vi "File.Search for Files or Folders, List Move or Copy.vi"(4 "Filter List":string, 6 "Destination Path":path, 7 "Files(F)/Folders(T)":bool, 8 "error in":errorcluster, 9 "Filters(Contain)":string[](array[string]), 10 "Action":enum16{"List", "Move", "Copy"}(ring), 11 "Source Paths":path[](array[path])) -> (0 "error out":errorcluster, 3 "Found Items":path[](array[path]))   [LabVIEW 2018]
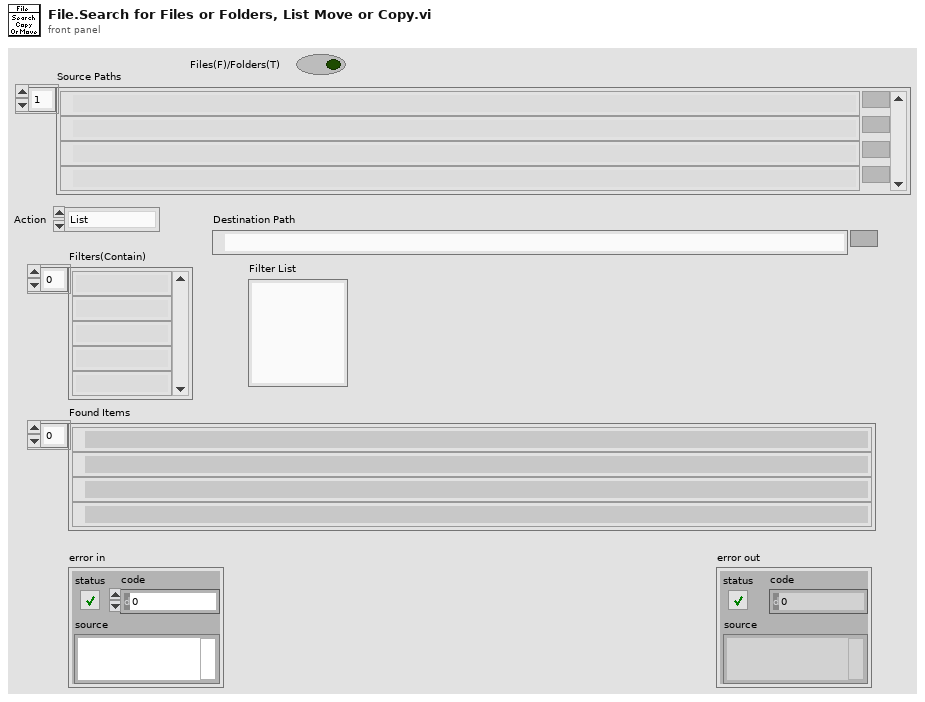
[diagram p1: front panel]
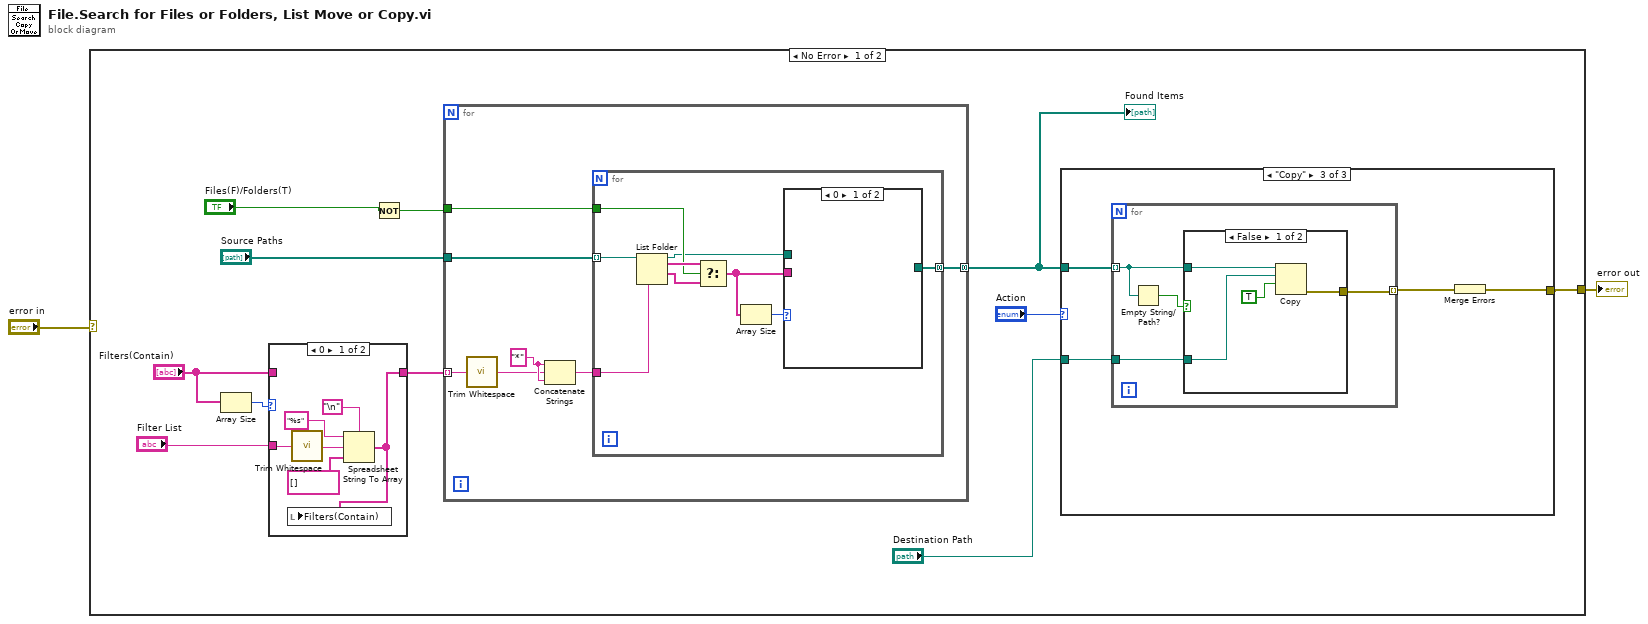
[diagram p0: block diagram]
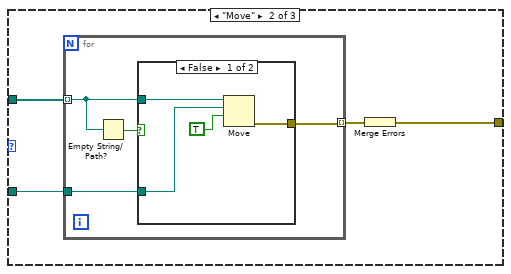
[diagram p4: hidden frame]
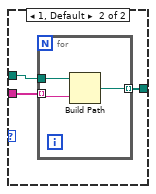
[diagram p7: hidden frame]
diagram:
  n1 = case shown="No Error" "error in" {
    selector: "error in" -> [_ w67]
    tunnel: [w9 w67] -> w2
    frame No Error {
      n2 = Array Size(array="Filters(Contain)") -> (size(s)=w7:i32)
      n3 = case shown="0" w7 {
        tunnel: "Filter List" -> [w19 _]
        tunnel: [w14 w20] -> w6
        tunnel: "Filters(Contain)" -> [_ w20]
        frame 0 {
          n4 = call <vilib>:"Trim Whitespace.vi"("string"=w19) -> ("trimmed string"=w18:string)  [unwired: 1 in]
          n5 = Spreadsheet String To Array(delimiter (Tab)="\n", format string="%s", spreadsheet string=w18, array type (2D Dbl)=string[] [] ("Filters(Contain)")) -> (array=w14:string[])
          n6 = local write "Filters(Contain)"(w14) -> ()
        }
        frame Default {
        }
      }
      n7 = Not(x="Files(F)/Folders(T)") -> (.not. x?=w4:bool)
      n8 = for {
        tunnel: "Source Paths" -> [w51]
        tunnel: w4 -> [w50]
        tunnel: w6 -> [w46] mode=indexing
        tunnel: [w47] -> w11 mode=concatenating
        w49 = "*"
        n9 = call <vilib>:"Trim Whitespace.vi"("string"=w46) -> ("trimmed string"=w45:string)  [unwired: 1 in]
        n10 = Concatenate Strings(w49, w45, w49) -> (w48:string)
        n11 = for {
          tunnel: w51 -> [w60] mode=indexing
          tunnel: w50 -> [w57]
          tunnel: w48 -> [w54]
          tunnel: [w55] -> w47 mode=concatenating
          n12 = List Folder(path=w60, pattern=w54) -> (path out=w56:path, filenames=w59:string[], folder names=w58:string[])  [unwired: 2 in, 1 out]
          n13 = Select(t=w59, s=w57, f=w58) -> (s? t:f=w53:string[])
          n14 = Array Size(array=w53) -> (size(s)=w52:i32)
          n15 = case shown="0" w52 {
            tunnel: w53 -> [_ w63]
            tunnel: w56 -> [_ w62]
            tunnel: [_ w61] -> w55
            frame 0 {
            }
            frame 1, Default {
              n16 = for {
                tunnel: w63 -> [w65] mode=indexing
                tunnel: w62 -> [w66]
                tunnel: [w64] -> w61 mode=indexing
                n17 = Build Path(base path=w66, name or relative path=w65) -> (appended path=w64:path)
              }
            }
          }
        }
      }
      "Found Items" <- w11
      n18 = case shown="\"Copy\"" "Action" {
        tunnel: w11 -> [_ w24 w36]
        tunnel: "Destination Path" -> [_ w23 w35]
        tunnel: [_ w21 w33] -> w9
        frame "List", Default {
          # "Do Nothing"
        }
        frame "Move" {
          n19 = for {
            tunnel: w24 -> [w26] mode=indexing
            tunnel: w23 -> [w28]
            tunnel: [w27] -> w22 mode=indexing
            n20 = Empty String/Path?(string/path=w26) -> (empty?=w25:bool)
            n21 = case shown="False" w25 {
              tunnel: w28 -> [w32 _]
              tunnel: [w30 _] -> w27
              tunnel: w26 -> [w29 _]
              frame False {
                n22 = Move(source path=w29, 9:TRUE ("overwrite (F)"), 10:w32) -> (error out=w30:errorcluster)  [unwired: 2 in, 2 out]
              }
              frame True {
              }
            }
          }
          n23 = Merge Errors(w22) -> (w21:errorcluster)
        }
        frame "Copy" {
          n24 = for {
            tunnel: w36 -> [w38] mode=indexing
            tunnel: w35 -> [w40]
            tunnel: [w39] -> w34 mode=indexing
            n25 = Empty String/Path?(string/path=w38) -> (empty?=w37:bool)
            n26 = case shown="False" w37 {
              tunnel: w40 -> [w44 _]
              tunnel: [w42 _] -> w39
              tunnel: w38 -> [w41 _]
              frame False {
                n27 = Copy(9:TRUE ("overwrite (F)"), 10:w44, 11:w41) -> (0:w42:errorcluster)  [unwired: 2 in, 2 out]
              }
              frame True {
              }
            }
          }
          n28 = Merge Errors(w34) -> (w33:errorcluster)
        }
      }
    }
    frame Error {
    }
  }
  "error out" <- w2
